vi "AutoShimmy.vi"   [LabVIEW 2014]
uses:
  Robot Global Data.vi
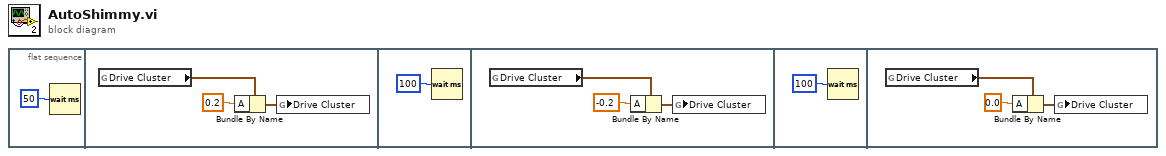
[diagram p0: block diagram]
diagram:
  n1 = flat-sequence {
    frame #0 {
      n2 = Wait (ms)(milliseconds to wait=u32 50) -> ()  [unwired: 1 out]
    }
    frame #1 {
      n3 = global read "Robot Global Data.vi" "Drive Cluster"() -> (w4:cluster{"A":dbl, "B":dbl, "R":dbl, "Gyro":dbl})
      n4 = Bundle By Name(cluster=w4, "A"=0.2) -> (w3:cluster{"A":dbl, "B":dbl, "R":dbl, "Gyro":dbl})
      n5 = global write "Robot Global Data.vi" "Drive Cluster"(w3) -> ()
    }
    frame #2 {
      n6 = Wait (ms)(milliseconds to wait=u32 100) -> ()  [unwired: 1 out]
    }
    frame #3 {
      n7 = global read "Robot Global Data.vi" "Drive Cluster"() -> (w6:cluster{"A":dbl, "B":dbl, "R":dbl, "Gyro":dbl})
      n8 = Bundle By Name(cluster=w6, "A"=-0.2) -> (w7:cluster{"A":dbl, "B":dbl, "R":dbl, "Gyro":dbl})
      n9 = global write "Robot Global Data.vi" "Drive Cluster"(w7) -> ()
    }
    frame #4 {
      n10 = Wait (ms)(milliseconds to wait=u32 100) -> ()  [unwired: 1 out]
    }
    frame #5 {
      n11 = global read "Robot Global Data.vi" "Drive Cluster"() -> (w12:cluster{"A":dbl, "B":dbl, "R":dbl, "Gyro":dbl})
      n12 = Bundle By Name(cluster=w12, "A"=0.0) -> (w11:cluster{"A":dbl, "B":dbl, "R":dbl, "Gyro":dbl})
      n13 = global write "Robot Global Data.vi" "Drive Cluster"(w11) -> ()
    }
  }
